vi "Connect Power Supply 2 to UUT.vi"(9 "Connect":bool, 11 "Device":string="Dev1") -> ()   [LabVIEW 2015]
panel:
  in  "error in":errorcluster
  out "error out":errorcluster={"status"=TRUE, "code"=-200220, "source"="DAQmx Create Channel (DO-Digital Output).vi:2<append>\n<B>Device Specified: </B>Dev1\n\n<B>Task Name: </B>_unnamedTask<0>"}
  out "Array":cluster{bool, string}[](array[cluster])
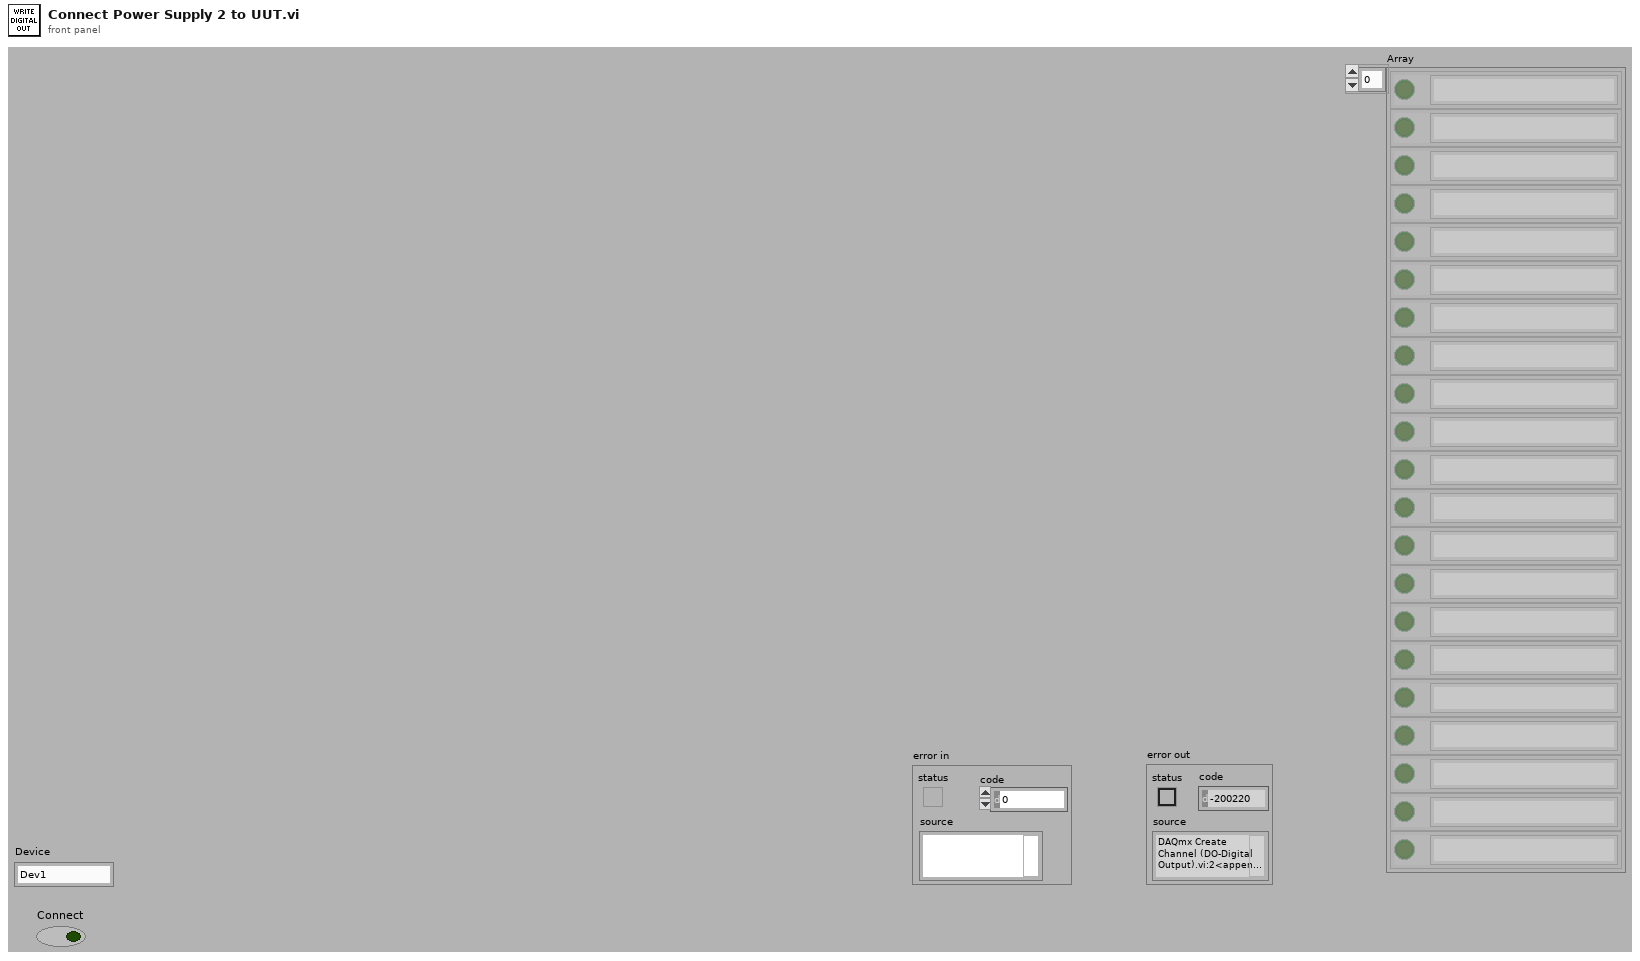
[diagram p1: front panel]
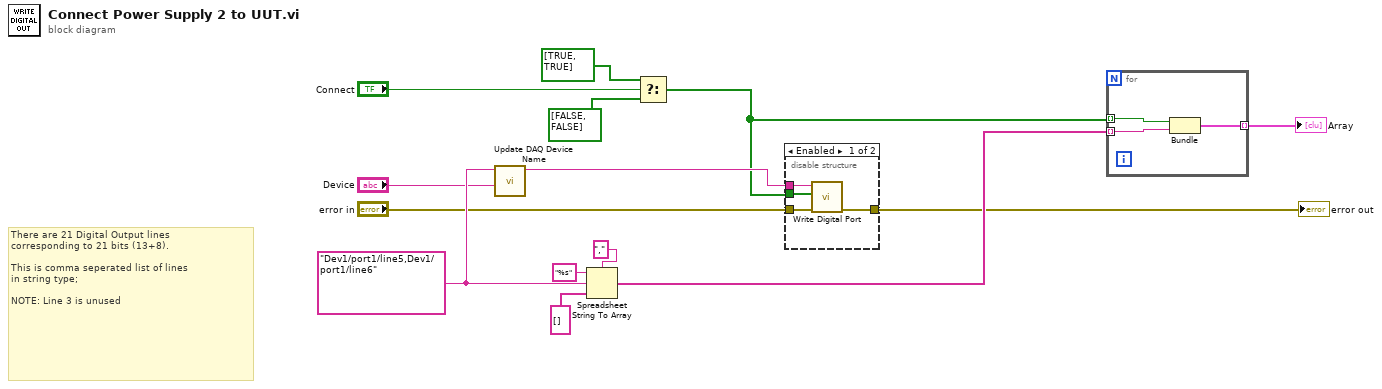
[diagram p0: block diagram]
diagram:
  w12 = "Dev1/port1/line5,Dev1/port1/line6" ("String")
  # "There are 21 Digital Output lines \ncorresponding to 21 bits (13+8).\n\nThis is comma seperated list of lines\nin string type;\n\nNOTE: Line 3 is unused"
  n1 = call "Update DAQ Device Name.vi"("Device Name"="Device", "Lines in (String)"=w12) -> ("Lines out (DAQmx Physical Channels)"=w8:tag)  [unwired: 9 in]
  n2 = Spreadsheet String To Array(delimiter (Tab)=",", format string="%s", spreadsheet string=w12, array type (2D Dbl)=string[] []) -> (array=w13:string[])
  n3 = Select(t=bool[] [TRUE, TRUE], s="Connect", f=bool[] [FALSE, FALSE]) -> (s? t:f=w1:bool[])
  n4 = disable-structure shown="Enabled" {
    disable-tunnel: "error in" -> [w18 _]
    disable-tunnel: [w17 _] -> w7
    disable-tunnel: w1 -> [w16 _]
    disable-tunnel: w8 -> [w15 _]
    frame Enabled {
      n5 = call "Write Digital Port.vi"("error in"=w18, "Data"=w16, "Line(s)"=w15) -> ("error out"=w17:errorcluster)  [unwired: 8 in]
    }
    frame Disabled {
    }
  }
  "error out" <- w7
  n6 = for {
    tunnel: w1 -> [w21] mode=indexing
    tunnel: w13 -> [w20] mode=indexing
    tunnel: [w19] -> w14 mode=indexing
    n7 = Bundle(w21, w20) -> (w19:cluster{bool, string})  [unwired: 1 in]
  }
  "Array" <- w14
